vi "Disconnect.vi"(8 "error in":errorcluster, 11 "Control Box in":refnum<class "Control Box.lvclass">) -> (0 "error out":errorcluster, 3 "Control Box out":refnum<class "Control Box.lvclass">)   [LabVIEW 2018, in "Control Box.lvlib" / "Control Box.lvclass"]
uses:
  Control Box.lvclass
  Control Box.lvclass/Control Box.ctl
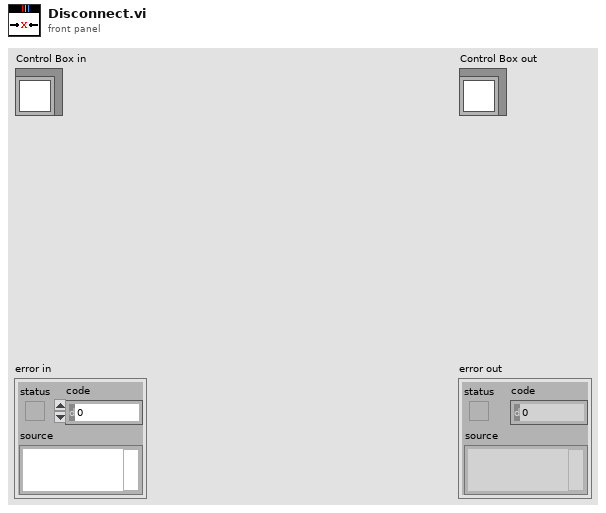
[diagram p1: front panel]
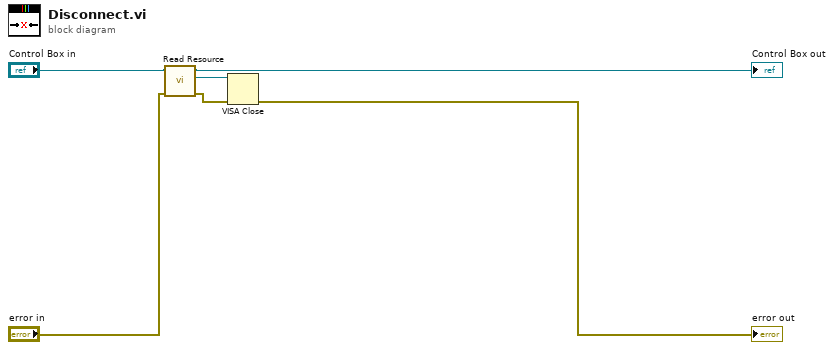
[diagram p0: block diagram]
diagram:
  n1 = call "Read Resource.vi"("error in (no error)"="error in", "Control Box in"="Control Box in") -> ("error out"=w3:errorcluster, "Resource"=w4:refnum<visa-resource-name>, "Control Box out"=→"Control Box out":refnum<class "Control Box.lvclass">)  [unwired: 7 in]
  n2 = VISA Close(VISA resource name=w4, error in (no error)=w3) -> (error out=→"error out":errorcluster)
